vi "Initialize USB.vi"(8 "error in":errorcluster, 11 "OphirFastX (in)":refnum<k7>) -> (0 "error out":errorcluster, 3 "OphirFastX (out)":refnum<k7>)   [LabVIEW 2009]
panel:
  # "Guillaume Plateau - yguig2@yahoo.fr"
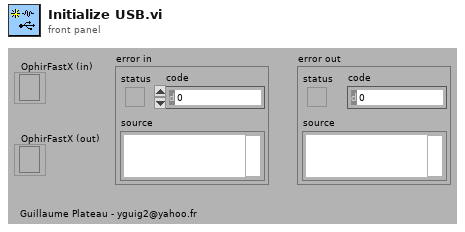
[diagram p1: front panel]
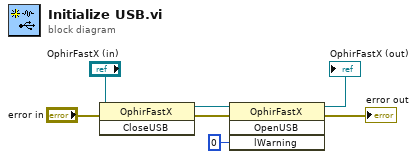
[diagram p0: block diagram]
diagram:
  n1 = invoke class="OphirFastX" method="CloseUSB"(reference="OphirFastX (in)", error in="error in") -> (reference out=w6:refnum<k7>, error out=w4:errorcluster)  [unwired: 1 in, 1 out]
  n2 = invoke class="OphirFastX" method="OpenUSB"(reference=w6, error in=w4, "lWarning"=0) -> (reference out=→"OphirFastX (out)":refnum<k7>, error out=→"error out":errorcluster)  [unwired: 1 in, 2 out]
